vi "OpticalFlowWorm.vi"() -> ()   [LabVIEW 2014]
uses:
  <vilib>/vision/NI_Vision_Development_Module.lvlib
panel:
  in  "Threshold":dbl=7.0
  in  "Step Size":i32=1 min=1
  out "Numeric":i32=75
  out "Image":T1(plugin-control)
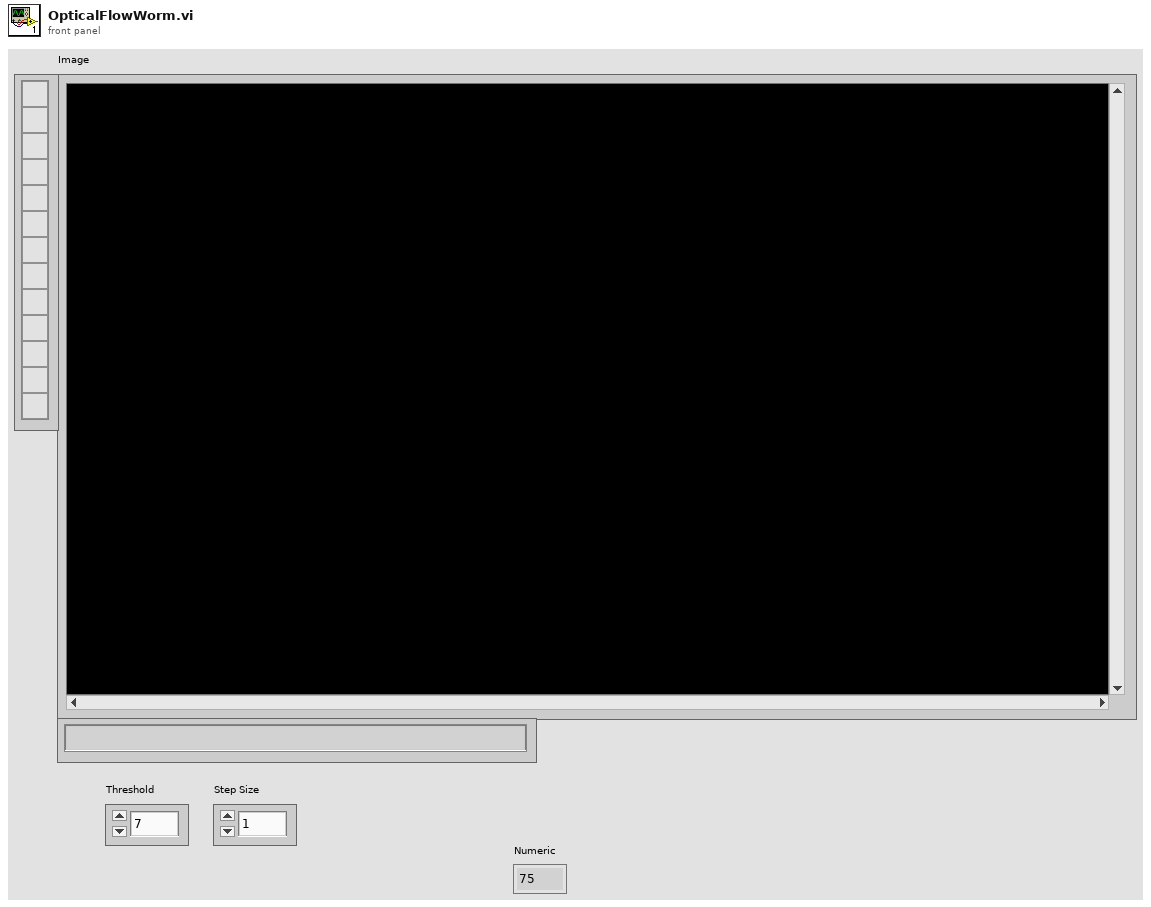
[diagram p1: front panel]
types:
  T1 = typedef "IMAQ Image.ctl" = refnum<image>
  T2 = typedef "IMAQ AVI2 Refnum.ctl" = refnum<k20>
  T3 = typedef "Image Type" = u32
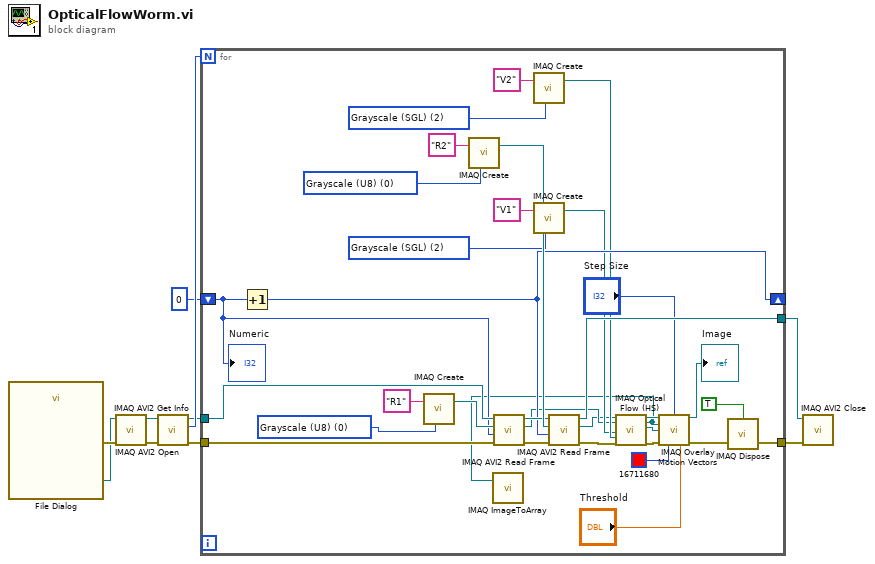
[diagram p0: block diagram]
diagram:
  n1 = call "File Dialog"() -> ("selected path"=w8:path, "error out"=w10:errorcluster)  [unwired: 12 in, 2 out]
  n2 = call "IMAQ AVI2 Open"("error in (no error)"=w10, "AVI File Path"=w8) -> ("error out"=w9:errorcluster, "AVI Refnum"=w7:T2)  [unwired: 8 in]
  n3 = call "IMAQ AVI2 Get Info"("error in (no error)"=w9, "AVI Refnum"=w7) -> ("error out"=w4:errorcluster, "Number of Frames"=w6:u32, "AVI Refnum (duplicate)"=w5:T2)  [unwired: 5 in, 2 out]
  n4 = for {
    N: w6 -> [_]
    tunnel: w5 -> [w43]
    tunnel: w4 -> [w42]
    tunnel: [w21] -> w3
    tunnel: [w32] -> w2
    shift-right: [w25] -> _
    shift-left: 0 -> [w26]
    w27 = T3 2 items=["Grayscale (U8)", "Grayscale (I16)", "Grayscale (SGL)", "Complex (CSG)", "RGB (U32)", "HSL (U32)", "RGB (U64)", "Grayscale (U16)"] ("Image Type")
    w28 = T3 2 items=["Grayscale (U8)", "Grayscale (I16)", "Grayscale (SGL)", "Complex (CSG)", "RGB (U32)", "HSL (U32)", "RGB (U64)", "Grayscale (U16)"] ("Image Type")
    w29 = T3 0 items=["Grayscale (U8)", "Grayscale (I16)", "Grayscale (SGL)", "Complex (CSG)", "RGB (U32)", "HSL (U32)", "RGB (U64)", "Grayscale (U16)"] ("Image Type")
    w30 = T3 0 items=["Grayscale (U8)", "Grayscale (I16)", "Grayscale (SGL)", "Complex (CSG)", "RGB (U32)", "HSL (U32)", "RGB (U64)", "Grayscale (U16)"] ("Image Type")
    n5 = Increment(x=w26) -> (x+1=w25:i32)
    n6 = call "IMAQ Create"("Image Name"="R1", "Image Type"=w30) -> ("New Image"=w40:T1)  [unwired: 3 in, 1 out]
    n7 = call "IMAQ Create"("Image Name"="R2", "Image Type"=w29) -> ("New Image"=w37:T1)  [unwired: 3 in, 1 out]
    n8 = call "IMAQ AVI2 Read Frame"("error in (no error)"=w42, "Frame Number"=w26, "Image"=w40, "AVI Refnum"=w43) -> ("error out"=w41:errorcluster, "Image Out"=w15:T1, "AVI Refnum (duplicate)"=w36:T2)  [unwired: 5 in]
    n9 = call "IMAQ Create"("Image Name"="V2", "Image Type"=w28) -> ("New Image"=w17:T1)  [unwired: 3 in, 1 out]
    n10 = call "IMAQ Create"("Image Name"="V1", "Image Type"=w27) -> ("New Image"=w16:T1)  [unwired: 3 in, 1 out]
    n11 = call "IMAQ AVI2 Read Frame"("error in (no error)"=w41, "Frame Number"=w25, "Image"=w37, "AVI Refnum"=w36) -> ("error out"=w19:errorcluster, "Image Out"=w14:T1, "AVI Refnum (duplicate)"=w32:T2)  [unwired: 5 in]
    n12 = call "IMAQ Optical Flow (HS)"("Current Frame"=w14, "Previous Frame"=w15, "Velocity Component 1 In"=w16, "Velocity Component 2 In"=w17, "error in (no error)"=w19) -> ("Current Frame Out (dup)"=w13:T1, "Velocity Component 1 Out"=w11:T1, "Velocity Component 2 Out"=w12:T1, "error out"=w18:errorcluster)  [unwired: 11 in]
    n13 = call "IMAQ ImageToArray"("Image"=w11) -> ()  [unwired: 3 in, 5 out]
    n14 = call "IMAQ Overlay Motion Vectors"("Image"=w13, "Step Size"="Step Size", "Velocity Component 1"=w11, "Velocity Component 2"=w12, "error in (no error)"=w18, "Color"=u32 16711680, "Threshold"="Threshold") -> ("Image Out"=→"Image":T1, "error out"=w22:errorcluster)  [unwired: 7 in]
    n15 = call "IMAQ Dispose"("All Images? (No)"=TRUE, "error in (no error)"=w22) -> ("error out"=w21:errorcluster)  [unwired: 4 in]
    "Numeric" <- w26
  }
  n16 = call "IMAQ AVI2 Close"("error in (no error)"=w3, "AVI Refnum"=w2) -> ()  [unwired: 9 in, 1 out]
